vi "Write Sub Panel Coin.vi"(8 "error in (no error)":errorcluster, 10 "Sub Panel Coin":refnum<vi>, 11 "Monedas USD in":refnum<class "Monedas USD.lvclass">) -> (0 "error out":errorcluster, 3 "Monedas USD out":refnum<class "Monedas USD.lvclass">)   [LabVIEW 2020, in "Monedas USD.lvlib" / "Monedas USD.lvclass"]
uses:
  Monedas USD.lvclass
  Monedas USD.lvclass/Monedas USD.ctl
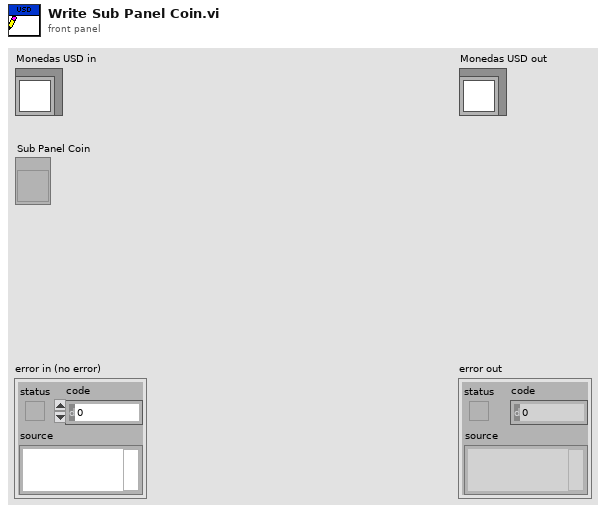
[diagram p1: front panel]
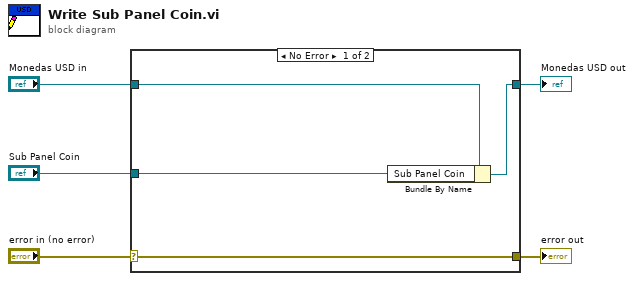
[diagram p0: block diagram]
diagram:
  n1 = case shown="No Error" "error in (no error)" {
    selector: "error in (no error)" -> [w9 w10]
    tunnel: [w9 w10] -> w4
    tunnel: [w7 w11] -> w2
    tunnel: "Monedas USD in" -> [w8 w11]
    tunnel: "Sub Panel Coin" -> [w6 _]
    frame No Error {
      n2 = Bundle By Name(cluster=w8, "Sub Panel Coin"=w6) -> (w7:refnum<class "Monedas USD.lvclass">)
    }
    frame Error {
    }
  }
  "error out" <- w4
  "Monedas USD out" <- w2
